vi "Calculate pretomo stack positions.vi"(8 "error in (no error)":errorcluster, 11 "Tomo in":refnum<class "Tomo.lvclass">) -> (0 "error out":errorcluster, 1 "Y pos":dbl[unit], 2 "X pos":dbl[unit], 3 "Tomo out":refnum<class "Tomo.lvclass">, 5 "Z pos":dbl[unit])   [LabVIEW 2012, in "Tomo.lvclass"]
uses:
  Tomo.lvclass
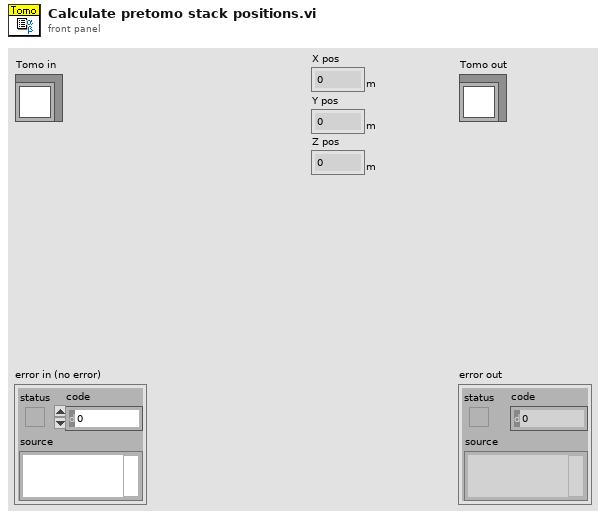
[diagram p1: front panel]
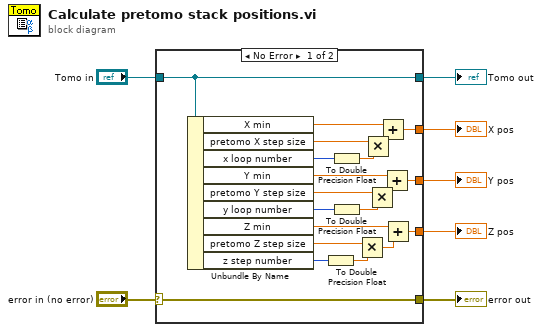
[diagram p0: block diagram]
diagram:
  n1 = case shown="No Error" "error in (no error)" {
    selector: "error in (no error)" -> [w27 w29]
    tunnel: [w27 w29] -> w6
    tunnel: [w26 w28] -> w4
    tunnel: "Tomo in" -> [w26 w28]
    tunnel: [w15 _] -> w3
    tunnel: [w14 _] -> w2
    tunnel: [w8 _] -> w1
    frame No Error {
      n2 = Unbundle By Name(w26) -> ("X min"=w21:dbl[unit], "pretomo X step size"=w22:dbl[unit], "x loop number"=w24:i32, "Y min"=w18:dbl[unit], "pretomo Y step size"=w17:dbl[unit], "y loop number"=w25:i32, "Z min"=w10:dbl[unit], "pretomo Z step size"=w11:dbl[unit], "z step number"=w13:i32)
      n3 = To Double Precision Float(number=w13) -> (double precision float=w12:dbl)
      n4 = To Double Precision Float(number=w24) -> (double precision float=w23:dbl)
      n5 = To Double Precision Float(number=w25) -> (double precision float=w16:dbl)
      n6 = Multiply(x=w11, y=w12) -> (x*y=w9:dbl[unit])
      n7 = Multiply(x=w22, y=w23) -> (x*y=w20:dbl[unit])
      n8 = Multiply(x=w17, y=w16) -> (x*y=w19:dbl[unit])
      n9 = Add(x=w21, y=w20) -> (x+y=w15:dbl[unit])
      n10 = Add(x=w18, y=w19) -> (x+y=w14:dbl[unit])
      n11 = Add(x=w10, y=w9) -> (x+y=w8:dbl[unit])
    }
    frame Error {
    }
  }
  "error out" <- w6
  "Tomo out" <- w4
  "X pos" <- w3
  "Y pos" <- w2
  "Z pos" <- w1
